vi "USBCamTest.vi"() -> ()   [LabVIEW 2020]
uses:
  <vilib>/userDefined/High Color/IMAQdx.ctl
  <vilib>/vision/driver/IMAQdx.llb/IMAQdx Acquisition Mode.ctl
  <vilib>/vision/driver/IMAQdx.llb/IMAQdx Buffer Number Mode.ctl
  <vilib>/vision/driver/NI_Vision_Acquisition_Software.lvlib
  <resource>/objmgr/imaqdx.rc
panel:
  in  "VideoMode":u32=10 max=15 step=1
  out "error out":errorcluster
  in  "stop":bool
  out "Acquired Frames/s":dbl
  out "Image":T1(plugin-control)
  in  "Session In":T2="cam1"
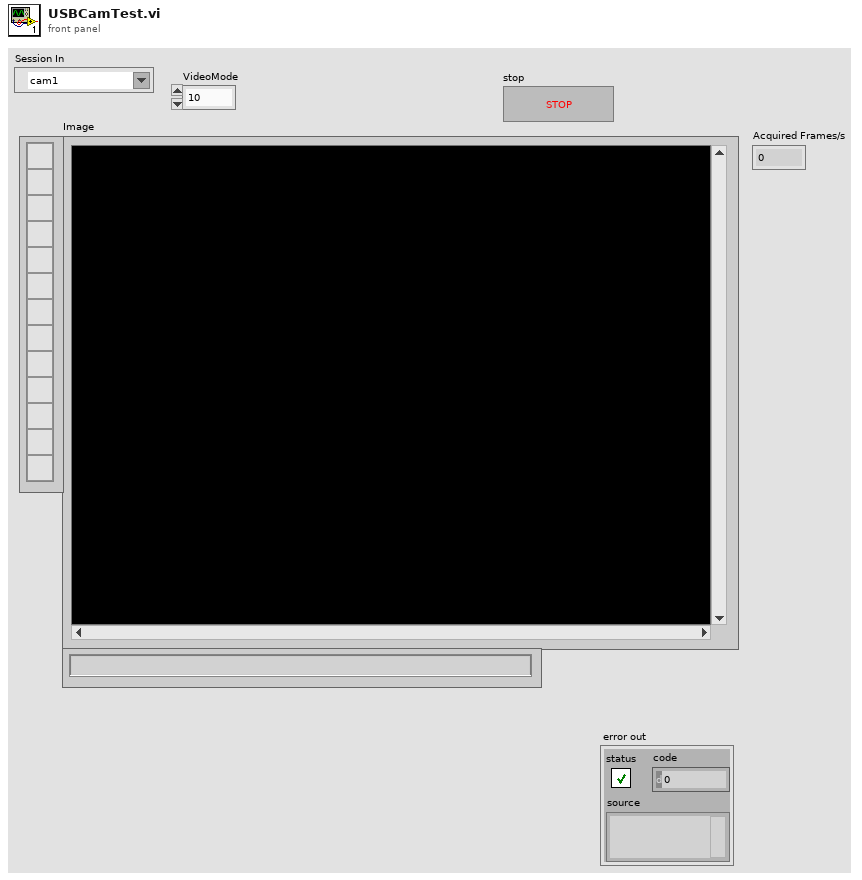
[diagram p1: front panel]
types:
  T1 = typedef "IMAQ Image.ctl" = refnum<image>
  T2 = typedef "IMAQdx.ctl" = refnum<k21>
  T3 = typedef "NI_Vision_Acquisition_Software.lvlib/IMAQdx Acquisition Mode.ctl" = enum32{"One Shot", "Continuous"}
  T4 = typedef "NI_Vision_Acquisition_Software.lvlib/IMAQdx Buffer Number Mode.ctl" = enum32{"Next", "Last", "Buffer Number", "Every", "Last New"}
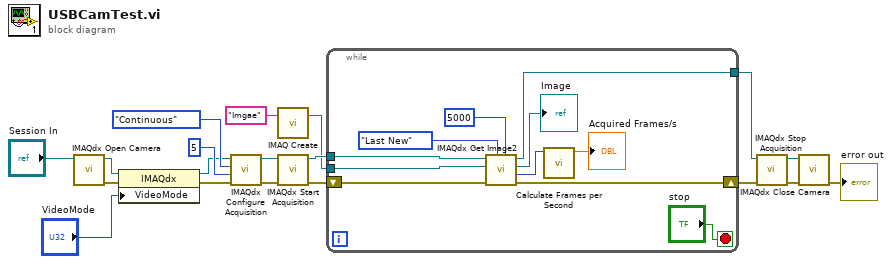
[diagram p0: block diagram]
diagram:
  n1 = call <vilib>:"IMAQdx Open Camera.vi"("Session In"="Session In") -> ("error out"=w4:errorcluster, "Session Out"=w5:T2)  [unwired: 9 in]
  n2 = property class="IMAQdx"(reference=w5, error in=w4, "VideoMode"="VideoMode") -> (reference out=w3:T2, error out=w2:errorcluster)
  n3 = call <vilib>:"IMAQdx Configure Acquisition.vi"("error in"=w2, "Number of Buffers"=u32 5, "Continuous?"=IMAQdx_Acquisition_Mode."Continuous", "Session In"=w3) -> ("error out"=w15:errorcluster, "Session Out"=w16:T2)  [unwired: 6 in]
  n4 = call "IMAQ Create"("Image Name"="Imgae") -> ("New Image"=w11:T1)  [unwired: 4 in, 1 out]
  n5 = call <vilib>:"IMAQdx Start Acquisition.vi"("error in"=w15, "Session In"=w16) -> ("error out"=w12:errorcluster, "Session Out"=w13:T2)  [unwired: 8 in]
  n6 = while {
    tunnel: w13 -> [w30]
    tunnel: w11 -> [w28]
    shift-right: [w24] -> w9
    shift-left: w12 -> [w29]
    tunnel: [w20] -> w10
    stop <- "stop" stop-if-true
    n7 = call <vilib>:"IMAQdx Get Image2.vi"("Timeout (ms)"=5000, "Buffer Number Mode (Next)"=IMAQdx_Buffer_Number_Mode."Last New", "error in"=w29, "Image In"=w28, "Session In"=w30) -> ("error out"=w24:errorcluster, "Buffer Number Out"=w23:u32, "Image Out"=→"Image":T1, "Session Out"=w20:T2)  [unwired: 3 in]
    n8 = call <vilib>:"Calculate Frames per Second.vi"("Buffer Number"=w23) -> ("Acquired Frames/s"=→"Acquired Frames/s":dbl)  [unwired: 8 in, 2 out]
  }
  n9 = call <vilib>:"IMAQdx Stop Acquisition.vi"("error in"=w9, "Session In"=w10) -> ("error out"=w7:errorcluster, "Session Out"=w8:T2)  [unwired: 8 in]
  n10 = call <vilib>:"IMAQdx Close Camera.vi"("error in"=w7, "Session In"=w8) -> ("error out"=→"error out":errorcluster)  [unwired: 9 in]
